vi "getTimeChannelFromXml.vi"(8 "error in (no error)":errorcluster, 10 "Xml":refnum<class "xmlNode.lvclass">, 11 "ScriptEvent in":refnum<class "ScriptEvent.lvclass">) -> (0 "error out":errorcluster, 2 "Xml":refnum<class "xmlNode.lvclass">, 3 "ScriptEvent out":refnum<class "ScriptEvent.lvclass">)   [LabVIEW 2009, in "Tools.lvlib" / "Scripting.lvlib" / "ScriptEvent.lvclass"]
uses:
  ScriptEvent.lvclass
  xmlNode/xmlNode.lvclass
  DatabaseHelpers/Database Objects/Channel/Channel.lvclass
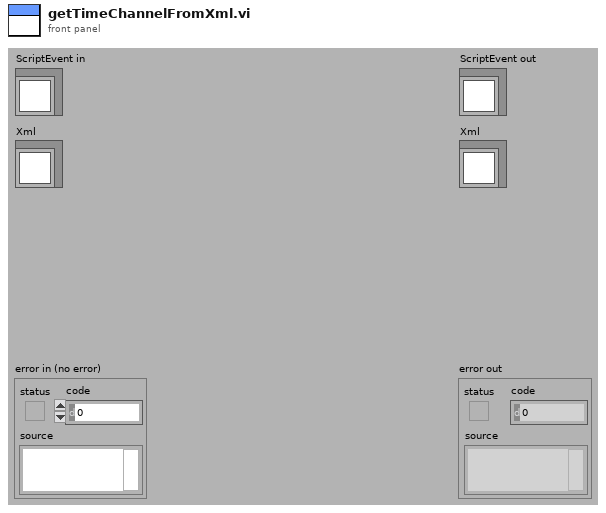
[diagram p1: front panel]
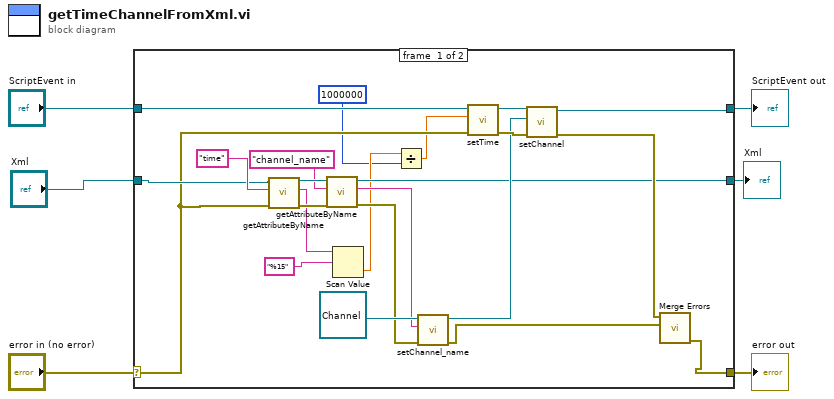
[diagram p0: block diagram]
diagram:
  n1 = case shown="No Error" "error in (no error)" {
    selector: "error in (no error)" -> [w14 w31]
    tunnel: [w13 w31] -> w5
    tunnel: [w17 w30] -> w3
    tunnel: "ScriptEvent in" -> [w19 w30]
    tunnel: "Xml" -> [w18 _]
    tunnel: [w12 _] -> w1
    frame #0 {
      n2 = call-dynamic "getAttributeByName.vi"("error in (no error)"=w14, "AttributeName"="time", "xmlNode in"=w18) -> ("error out"=w28:errorcluster, "attribute string"=w11:string, "xmlNode out"=w27:refnum<class "xmlNode.lvclass">)  [unwired: 6 in]
      n3 = call-dynamic "getAttributeByName.vi"("error in (no error)"=w28, "AttributeName"="channel_name", "xmlNode in"=w27) -> ("error out"=w20:errorcluster, "attribute string"=w24:string, "xmlNode out"=w12:refnum<class "xmlNode.lvclass">)  [unwired: 6 in]
      n4 = Scan Value(string=w11, format string="%15") -> (value=w9:dbl)  [unwired: 1 in, 1 out]
      n5 = Divide(x=w9, y=1000000) -> (x/y=w7:dbl)
      n6 = call "setChannel_name.vi"("error in (no error)"=w20, "channel_name"=w24, "Channel.lvclass in"=refnum<class "Channel.lvclass"> refnum ("Tools.lvlib:DatabaseHelpers.lvlib:Channel.lvclass")) -> ("error out"=w15:errorcluster, "Channel.lvclass out"=w21:refnum<class "Channel.lvclass">)  [unwired: 7 in]
      n7 = call "setTime.vi"("error in (no error)"=w14, "time"=w7, "ScriptEvent.lvclass in"=w19) -> ("error out"=w22:errorcluster, "ScriptEvent.lvclass out"=w23:refnum<class "ScriptEvent.lvclass">)  [unwired: 7 in]
      n8 = call-dynamic "setChannel.vi"("error in (no error)"=w22, "Channel.lvclass"=w21, "ScriptEvent.lvclass in"=w23) -> ("error out"=w16:errorcluster, "ScriptEvent.lvclass out"=w17:refnum<class "ScriptEvent.lvclass">)  [unwired: 7 in]
      n9 = call <vilib>:"Merge Errors.vi"("error in 2 (no error)"=w15, "error in 1 (no error)"=w16) -> ("error out"=w13:errorcluster)  [unwired: 5 in]
    }
    frame #1 {
    }
  }
  "error out" <- w5
  "ScriptEvent out" <- w3
  "Xml" <- w1
